vi "Initialise.vi"(8 "error in (no error)":errorcluster, 10 "Message in":refnum<class "InitialiseMessage.lvclass">, 11 "StageSPIM in":refnum<class "StageSPIM.lvclass">) -> (0 "error out":errorcluster, 3 "StageSPIM out":refnum<class "StageSPIM.lvclass">)   [LabVIEW 2012, in "StageSPIM.lvclass"]
doc: "This method is called when an initialise message is received. It mainly initialises the RabbitMQ connectivity. \n\nOverride this method when your component needs special initialisation (e.g. of software or hardware resources). In that case, don't forget to call the parent for proper implementation. If your component owns subcomponents, they count as resources, so you have to initialise them by calling their own initialise functions"
uses:
  StageSPIM.lvclass
  <vilib>/Distrio/Murmex/InitialiseMessage/InitialiseMessage.lvclass
  <vilib>/Distrio/Murmex/Murmex/Murmex.lvclass
  StageSPIM.lvclass/StageSPIM.ctl
panel:
  # "This method is called when the INTIALISE\ntrigger is sent. \n\nOverride this method when your component needs to\nrespond to this trigger. \n\nCall parent for proper implementation"
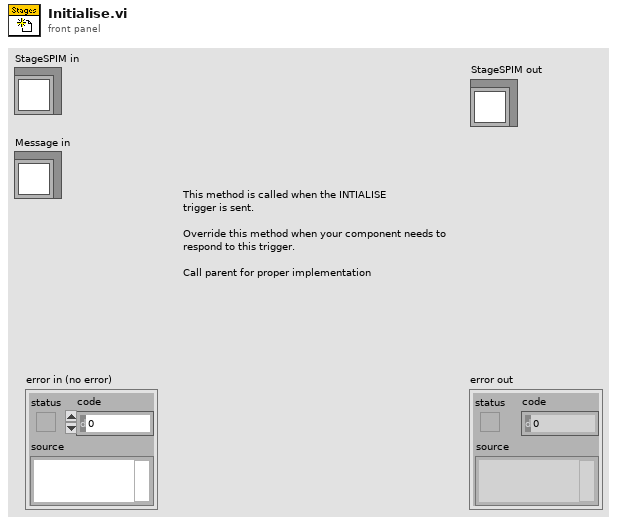
[diagram p1: front panel]
types:
  T1 = cluster{"Register DC":bool, "DaisyChain Search?":bool, "Device ID":i32}[][]
  T2 = cluster{"RON Affected axes":string[], "Reference mode":bool[], "Check FRF?":bool}
  T3 = typedef "StageSPIM.lvclass/port_control.ctl" = i32
  T4 = typedef "StageSPIM.lvclass/baud_rate_control.ctl" = u16
  T5 = typedef "StageSPIM.lvclass/connection_type.ctl" = enum16{"RS232", "RS232 DaisyChain", "USB", "USB_DaisyChain"}
  T6 = cluster{"Register DC":bool, "DaisyChain Search?":bool, "Device ID":i32}
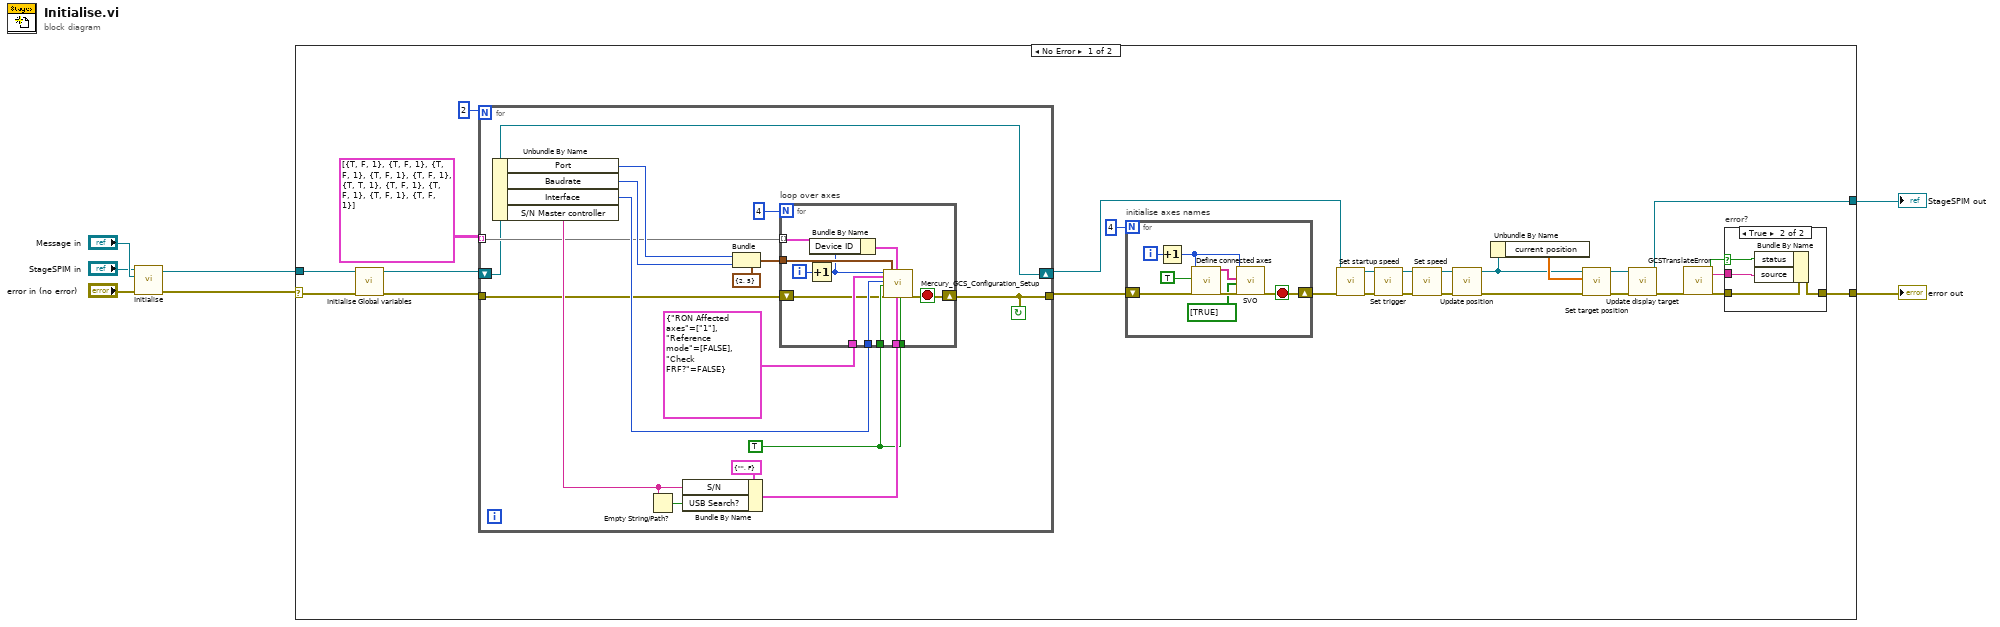
[diagram p0: block diagram]
diagram:
  n1 = call-parent "Initialise.vi"("error in (no error)"="error in (no error)", "Message in"="Message in", "Murmex in"="StageSPIM in") -> ("error out"=w4:errorcluster, "Murmex out"=w3:refnum<class "StageSPIM.lvclass">)  [unwired: 7 in]
  n2 = case shown="No Error" w4 {
    selector: w4 -> [w25 w77]
    tunnel: w3 -> [w23 w76]
    tunnel: [w14 w76] -> w2
    tunnel: [w26 w77] -> w1
    frame No Error {
      n3 = call-dynamic "Initialise Global variables.vi"("error in (no error)"=w25, "StageSPIM in"=w23) -> ("error out"=w24:errorcluster, "StageSPIM out"=w22:refnum<class "StageSPIM.lvclass">)  [unwired: 8 in]
      n4 = for {
        N: 2 -> [_]
        tunnel: [w36] -> w29
        tunnel: w24 -> [w39]
        tunnel: T1 [[{"Register DC"=TRUE, "DaisyChain Search?"=FALSE, "Device ID"=1}, {"Register DC"=TRUE, "DaisyChain Search?"=FALSE, "Device ID"=1}, {"Register DC"=TRUE, "DaisyChain Search?"=FALSE, "Device ID"=1}, {"Register DC"=TRUE, "DaisyChain Search?"=FALSE, "Device ID"=1}, {"Register DC"=TRUE, "DaisyChain Search?"=FALSE, "Device ID"=1}], [{"Register DC"=TRUE, "DaisyChain Search?"=TRUE, "Device ID"=1}, {"Register DC"=TRUE, "DaisyChain Search?"=FALSE, "Device ID"=1}, {"Register DC"=TRUE, "DaisyChain Search?"=FALSE, "Device ID"=1}, {"Register DC"=TRUE, "DaisyChain Search?"=FALSE, "Device ID"=1}, {"Register DC"=TRUE, "DaisyChain Search?"=FALSE, "Device ID"=1}]] -> [w38] mode=indexing
        shift-right: [w37] -> w11
        shift-left: w22 -> [w37]
        stop <- w36 continue-if-true
        w44 = TRUE ("Switch servo on?")
        n5 = Unbundle By Name(w37) -> ("Port"=w42:T3, "Baudrate"=w41:T4, "Interface"=w40:T5, "S/N Master controller"=w46:string)
        n6 = Empty String/Path?(string/path=w46) -> (empty?=w47:bool)
        n7 = Bundle By Name(cluster=cluster{"S/N":string, "USB Search?":bool} {"S/N"="", "USB Search?"=FALSE} ("USB settings"), "S/N"=w46, "USB Search?"=w47) -> (w45:cluster{"S/N":string, "USB Search?":bool})
        n8 = Bundle(cluster=cluster{"Portnumber":i32, "Baudrate":u16} {"Portnumber"=2, "Baudrate"=5} ("RS232 settings"), "Portnumber"=w42, "Baudrate"=w41) -> (w49:cluster{"Portnumber":i32, "Baudrate":u16})
        n9 = for "loop over axes" {
          N: 4 -> [_]
          tunnel: w38 -> [w55] mode=indexing
          tunnel: w40 -> [w62]
          tunnel: w44 -> [w57]
          tunnel: w49 -> [w61]
          tunnel: T2 {"RON Affected axes"=["1"], "Reference mode"=[FALSE], "Check FRF?"=FALSE} ("RON settings") -> [w60]
          tunnel: w45 -> [w59]
          shift-right: [w58] -> w36
          shift-left: w39 -> [w52]
          tunnel: w44 -> [w56]
          i -> [w51]
          stop <- w58 stop-if-true
          n10 = Increment(x=w51) -> (x+1=w53:i32)
          n11 = Bundle By Name(cluster=w55, "Device ID"=w53) -> (w54:T6)
          n12 = call "Mercury_GCS_Configuration_Setup.vi"("System no."=w53, "RON settings"=w60, "Interface"=w62, "All axes?"=w56, "error in"=w52, "RS232 settings"=w61, "DaisyChain settings"=w54, "USB settings"=w59, "Switch servo on?"=w57) -> ("error out"=w58:errorcluster)  [unwired: 4 in, 6 out]
        }
      }
      n13 = for "initialise axes names" {
        N: 4 -> [_]
        shift-right: [w68] -> w13
        shift-left: w29 -> [w75]
        i -> [w73]
        stop <- w68 stop-if-true
        n14 = Increment(x=w73) -> (x+1=w69:i32)
        n15 = call "Define connected axes.vi"("System no."=w69, "Read from\ncontroller?"=TRUE ("Read from\ncontroller?"), "error in"=w75) -> ("Conn. Axes out"=w70:string[], "error out"=w72:errorcluster)  [unwired: 15 in]
        n16 = call "SVO.vi"("System no."=w69, "Axes to command"=w70, "Servo mode"=bool[] [TRUE], "error in"=w72) -> ("error out"=w68:errorcluster)  [unwired: 15 in]
      }
      n17 = call-dynamic "Set startup speed.vi"("error in (no error)"=w13, "StageSPIM in"=w11) -> ("error out"=w12:errorcluster, "StageSPIM out"=w9:refnum<class "StageSPIM.lvclass">)  [unwired: 8 in]
      n18 = call-dynamic "Set trigger.vi"("error in (no error)"=w12, "StageSPIM in"=w9) -> ("error out"=w10:errorcluster, "StageSPIM out"=w8:refnum<class "StageSPIM.lvclass">)  [unwired: 8 in]
      n19 = call-dynamic "Set speed.vi"("error in (no error)"=w10, "StageSPIM in"=w8) -> ("error out"=w27:errorcluster, "StageSPIM out"=w20:refnum<class "StageSPIM.lvclass">)  [unwired: 8 in]
      n20 = call-dynamic "Update position.vi"("error in (no error)"=w27, "StageSPIM in"=w20) -> ("error out"=w21:errorcluster, "StageSPIM out"=w16:refnum<class "StageSPIM.lvclass">)  [unwired: 8 in]
      n21 = Unbundle By Name(w16) -> ("current position"=w17:dbl[])
      n22 = call-dynamic "Set target position.vi"("error in (no error)"=w21, "target position"=w17, "StageSPIM in"=w16) -> ("error out"=w19:errorcluster, "StageSPIM out"=w15:refnum<class "StageSPIM.lvclass">)  [unwired: 7 in]
      n23 = call-dynamic "Update display target.vi"("error in (no error)"=w19, "StageSPIM in"=w15) -> ("error out"=w18:errorcluster, "StageSPIM out"=w14:refnum<class "StageSPIM.lvclass">)  [unwired: 8 in]
      n24 = call "GCSTranslateError.vi"("error in"=w18) -> ("GCS Error?"=w34:bool, "Error Description"=w32:string, "error out"=w33:errorcluster)  [unwired: 16 in]
      n25 = case "error?" shown="True" w34 {
        selector: w34 -> [_ w66]
        tunnel: w33 -> [w63 w67]
        tunnel: w32 -> [_ w65]
        tunnel: [w63 w64] -> w26
        frame False {
        }
        frame True {
          n26 = Bundle By Name(cluster=w67, "status"=w66, "source"=w65) -> (w64:errorcluster)
        }
      }
    }
    frame Error {
    }
  }
  "error out" <- w1
  "StageSPIM out" <- w2
